vi "new auto.vi"   [LabVIEW 2011]
uses:
  Robot Global Data.vi
types:
  T1 = typedef "WPI_MotorControlDeviceRef.ctl" = cluster{"DeviceStatus":errorcluster, "Type":enum16{"PWM", "CAN"}, "PWM":cluster{"Digital Module":T2, "PWM Channel":T3, "DeadBand":T4}, "CAN":cluster{"Device Number":u8, "Control Mode":T5, "Semaphore":T6, "Max Vout":dbl}, "Invert":bool, "TransformRef":T7, "InvTransformRef":T7}
  T2 = typedef "FPGA_TypedefDigitalModule.ctl" = enum16{"Digital Module 1", "Digital Module 2"}
  T3 = typedef "FPGA_DIOPWMChannel.ctl" = enum8{"PWM 1", "PWM 2", "PWM 3", "PWM 4", "PWM 5", "PWM 6", "PWM 7", "PWM 8", "PWM 9", "PWM 10", "Invalid"}
  T4 = typedef "WPI_PWMDeadband.ctl" = cluster{"Name":string, "maxPositivePwm":i32, "minPositivePwm":i32, "centerPwm":i32, "maxNegativePwm":i32, "minNegativePwm":i32, "angularRange":u16}
  T5 = typedef "WPI_CANJaguar_ControlMode.ctl" = enum8{"Percent VBus", "Current", "Speed", "Position", "Voltage"}
  T6 = typedef "Semaphore RefNum" = refnum<k1>
  T7 = typedef "WPI_PWMTransform_ConPane.ctl" = refnum<vi>
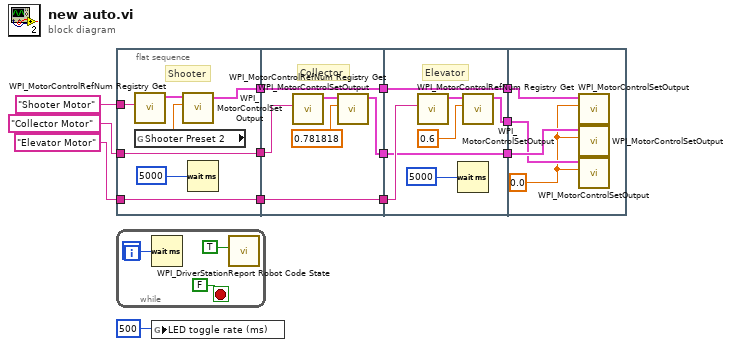
[diagram p0: block diagram]
diagram:
  n1 = flat-sequence {
    tunnel: "Shooter Motor" ("refnum name") -> [w19]
    tunnel: [w16] -> w13
    tunnel: "Collector Motor" ("refnum name") -> [w16]
    tunnel: "Elevator Motor" ("refnum name") -> [w15]
    tunnel: [w15] -> w12
    tunnel: [w14] -> w11
    tunnel: w13 -> [w24]
    tunnel: w12 -> [w23]
    tunnel: [w23] -> w10
    tunnel: w11 -> [w22]
    tunnel: [w22] -> w9
    tunnel: [w21] -> w8
    tunnel: w10 -> [w31]
    tunnel: w9 -> [w29]
    tunnel: [w29] -> w7
    tunnel: w8 -> [w28]
    tunnel: [w28] -> w6
    tunnel: [w27] -> w5
    tunnel: w7 -> [w37]
    tunnel: w6 -> [w36]
    tunnel: w5 -> [w35]
    frame #0 {
      # "Shooter"
      n2 = call <vilib>:"WPI_MotorControlRefNum Registry Get.vi"("refnum name"=w19) -> ("MotorControlDevRef"=w18:T1)  [unwired: 9 in, 1 out]
      n3 = global read "Robot Global Data.vi" "Shooter Preset 2"() -> (w20:dbl)
      n4 = call <vilib>:"WPI_MotorControlSetOutput.vi"("Output"=w20, "MotorControlDevRef"=w18) -> ("MotorControlDevRef"=w14:T1)  [unwired: 8 in, 1 out]
      n5 = Wait (ms)(milliseconds to wait=5000) -> ()  [unwired: 1 out]
    }
    frame #1 {
      # "Collector"
      n6 = call <vilib>:"WPI_MotorControlRefNum Registry Get.vi"("refnum name"=w24) -> ("MotorControlDevRef"=w26:T1)  [unwired: 9 in, 1 out]
      n7 = call <vilib>:"WPI_MotorControlSetOutput.vi"("Output"=0.781818, "MotorControlDevRef"=w26) -> ("MotorControlDevRef"=w21:T1)  [unwired: 8 in, 1 out]
    }
    frame #2 {
      # "Elevator"
      n8 = call <vilib>:"WPI_MotorControlRefNum Registry Get.vi"("refnum name"=w31) -> ("MotorControlDevRef"=w33:T1)  [unwired: 9 in, 1 out]
      n9 = Wait (ms)(milliseconds to wait=5000) -> ()  [unwired: 1 out]
      n10 = call <vilib>:"WPI_MotorControlSetOutput.vi"("Output"=0.6, "MotorControlDevRef"=w33) -> ("MotorControlDevRef"=w27:T1)  [unwired: 8 in, 1 out]
    }
    frame #3 {
      w34 = 0.0 ("Output")
      n11 = call <vilib>:"WPI_MotorControlSetOutput.vi"("Output"=w34, "MotorControlDevRef"=w37) -> ()  [unwired: 8 in, 2 out]
      n12 = call <vilib>:"WPI_MotorControlSetOutput.vi"("Output"=w34, "MotorControlDevRef"=w36) -> ()  [unwired: 8 in, 2 out]
      n13 = call <vilib>:"WPI_MotorControlSetOutput.vi"("Output"=w34, "MotorControlDevRef"=w35) -> ()  [unwired: 8 in, 2 out]
    }
  }
  n14 = while {
    stop <- FALSE stop-if-true
    n15 = Wait (ms)(milliseconds to wait=u32 20) -> ()  [unwired: 1 out]
    n16 = call <vilib>:"WPI_DriverStationReport Robot Code State.vi"("Autonomous"=TRUE) -> ()  [unwired: 10 in, 1 out]
  }
  n17 = global write "Robot Global Data.vi" "LED toggle rate (ms)"(u32 500 ("LED ms toggle rate")) -> ()
